vi "CumulativeArray.vi"(2 "error in":errorcluster, 3 "ArrayIn":u32[](array[numeric])) -> (0 "error out":errorcluster, 1 "ArrayOut":u32[](array[numeric]))   [LabVIEW 2014]
doc: "Use this template to build a VI to use as a subVI."
panel:
  # ":: MVi Framework V1.0 ::\nAuthor:Gaoke Yang\nEmail: gaoke.yang@yahoo.com\nWeb: www.mvicontrol.com\nCopyright (C) 2015, MVI Technologies All Rights Reserved"
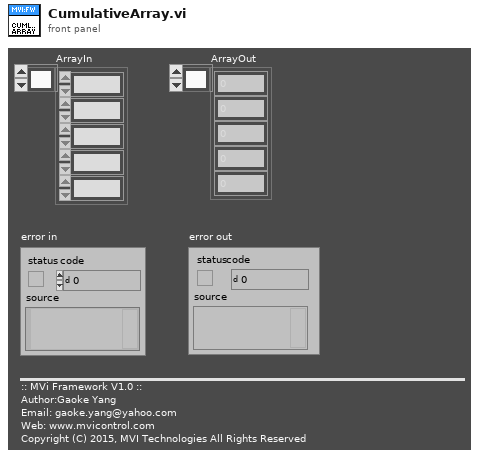
[diagram p1: front panel]
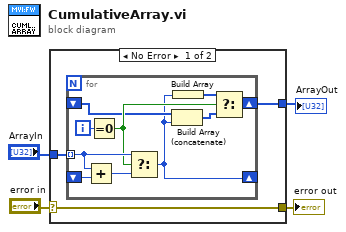
[diagram p0: block diagram]
diagram:
  n1 = case shown="No Error" "error in" {
    selector: "error in" -> [w7 w19]
    tunnel: [w7 w19] -> w3
    tunnel: [w6 w18] -> w2
    tunnel: "ArrayIn" -> [w5 w18]
    frame No Error {
      n2 = for {
        shift-right: [w10] -> _
        shift-left: _ -> [w15]
        tunnel: w5 -> [w14] mode=indexing
        shift-right: [w8] -> w6
        shift-left: _ -> [w11]
        i -> [w17]
        n3 = Add(x=w14, y=w15) -> (x+y=w16:u32)
        n4 = Equal To 0?(x=w17) -> (x = 0?=w13:bool)
        n5 = Select(t=w14, s=w13, f=w16) -> (s? t:f=w10:u32)
        n6 = Build Array (concatenate)(w11, w10) -> (w9:u32[])
        n7 = Build Array(w10) -> (w12:u32[])
        n8 = Select(t=w12, s=w13, f=w9) -> (s? t:f=w8:u32[])
      }
    }
    frame Error {
    }
  }
  "error out" <- w3
  "ArrayOut" <- w2
